vi "Config Curve Header.vi"(0 "VISA resource name":refnum<visa-resource-name>, 1 "Curve Data Format (0: mV/K)":u16(ring) items=["mV/K", "V/K", "Ohms/K", "Log Ohms/K", "Log Ohms/Log K"], 2 "Temp Coefficient (0: Negative)":u16(ring) items=["Negative", "Positive"], 5 "Curve (21)":dbl=21.0 min=21.0 max=60.0 step=1.0, 7 "Curve Name (\"\")":string, 9 "Curve Serial Number (\"\")":string, 11 "error in (no error)":errorcluster, 12 "Limit Value (0.000)":dbl min=0.0 max=1500.0 step=0.001 format="%.3f") -> (4 "VISA resource name out":refnum<visa-resource-name>, 15 "error out":errorcluster)   [LabVIEW 2019, in "Lake Shore Cryotronics 340.lvlib"]
doc: "This VI Configures a user curve header. Curves are not permanently updated in the curve FLASH until a Save Curve command has been issued using the LSCI 340 Save Curve to Flash.vi"
uses:
  Lake Shore Cryotronics 340.lvlib
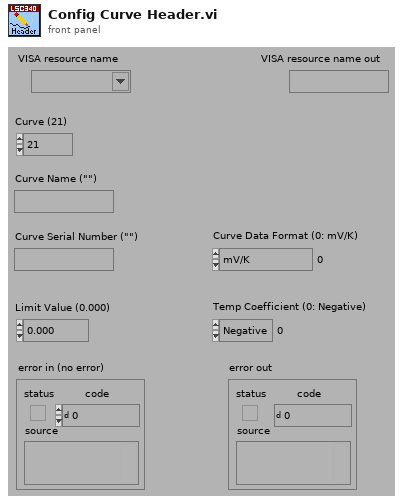
[diagram p1: front panel]
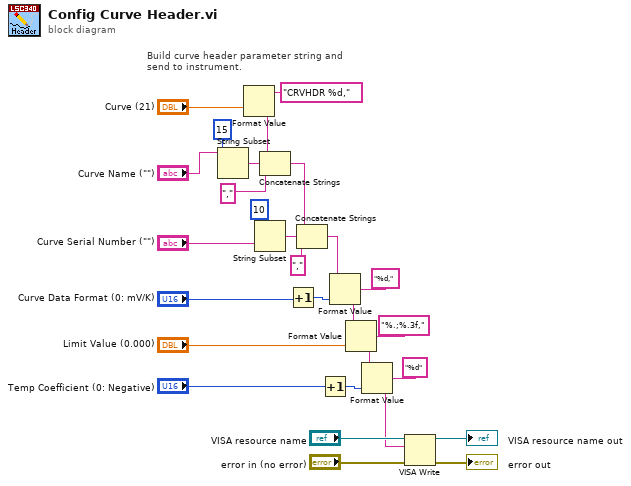
[diagram p0: block diagram]
diagram:
  # "Build curve header parameter string and\nsend to instrument."
  n1 = String Subset(string="Curve Name (\"\")", length (rest)=15) -> (substring=w22:string)  [unwired: 1 in]
  n2 = Format Value(format string="CRVHDR %d,", value (0)="Curve (21)") -> (output string=w23:string)  [unwired: 1 in]
  n3 = String Subset(string="Curve Serial Number (\"\")", length (rest)=10) -> (substring=w26:string)  [unwired: 1 in]
  n4 = Concatenate Strings(w23, w22, ",") -> (w27:string)
  n5 = Increment(x="Curve Data Format (0: mV/K)") -> (x+1=w17:u16)
  n6 = Concatenate Strings(w27, w26, ",") -> (w13:string)
  n7 = Increment(x="Temp Coefficient (0: Negative)") -> (x+1=w11:u16)
  n8 = Format Value(string ("")=w13, format string="%d,", value (0)=w17) -> (output string=w15:string)
  n9 = Format Value(string ("")=w15, format string="%.;%.3f,", value (0)="Limit Value (0.000)") -> (output string=w9:string)
  n10 = Format Value(string ("")=w9, format string="%d", value (0)=w11) -> (output string=w1:string)
  n11 = VISA Write(VISA resource name="VISA resource name", write buffer=w1, error in (no error)="error in (no error)") -> (VISA resource name out=→"VISA resource name out":refnum<visa-resource-name>, error out=→"error out":errorcluster)  [unwired: 1 out]
